vi "Configure Phase.vi"(0 "VISA resource name":refnum<visa-resource-name>, 5 "Phase Mode (0: Fixed)":i32(ring) items=["Fixed", "Step", "Pulse", "List"], 7 "Phase (0°)":dbl, 9 "Triggered Phase (0°)":dbl, 11 "error in (no error)":errorcluster) -> (4 "VISA resource name out":refnum<visa-resource-name>, 15 "error out":errorcluster)   [LabVIEW 2013, in "Cal Inst.lvlib" / "California Instruments iX Series.lvlib"]
doc: "Configures the output phases of the AC source. \n\n<b>Note:</b>\nWhen used on a single phase unit, the only discernible effect in using the phase commands is to cause an instantaneous shift in the output waveform phase."
uses:
  California Instruments iX Series.lvlib
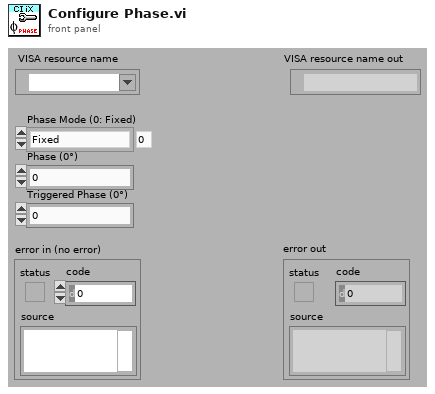
[diagram p1: front panel]
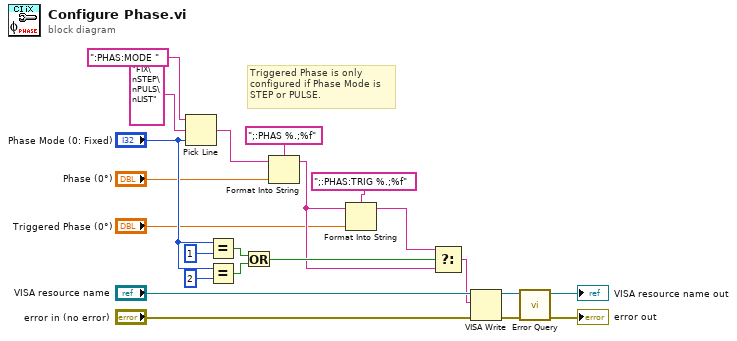
[diagram p0: block diagram]
diagram:
  # "Triggered Phase is only configured if Phase Mode is STEP or PULSE."
  n1 = Pick Line(string ("")=":PHAS:MODE ", multi-line string="FIX\nSTEP\nPULS\nLIST", line index="Phase Mode (0: Fixed)") -> (output string=w14:string)
  n2 = Equal?(x="Phase Mode (0: Fixed)", y=1) -> (x = y?=w9:bool)
  n3 = Equal?(x="Phase Mode (0: Fixed)", y=2) -> (x = y?=w8:bool)
  n4 = Or(x=w9, y=w8) -> (x .or. y?=w7:bool)
  n5 = Format Into String(format string=";:PHAS %.;%f", initial string=w14, "Phase (0°)") -> (resulting string=w6:string)  [unwired: 1 in, 1 out]
  n6 = Format Into String(format string=";:PHAS:TRIG %.;%f", initial string=w6, "Triggered Phase (0°)") -> (resulting string=w5:string)  [unwired: 1 in, 1 out]
  n7 = Select(t=w5, s=w7, f=w6) -> (s? t:f=w1:string)
  n8 = VISA Write(VISA resource name="VISA resource name", write buffer=w1, error in (no error)="error in (no error)") -> (VISA resource name out=w20:refnum<visa-resource-name>, error out=w19:errorcluster)  [unwired: 1 out]
  n9 = call "Error Query.vi"("error in (no error)"=w19, "VISA resource name"=w20) -> ("error out"=→"error out":errorcluster, "VISA resource name out"=→"VISA resource name out":refnum<visa-resource-name>)  [unwired: 6 in, 2 out]
